vi "Update_DATA.vi"(8 "error in (no error)":errorcluster, 10 "Name":string, 11 "HIS in":refnum<class "HIS.lvclass">) -> (0 "error out":errorcluster, 3 "HIS out":refnum<class "HIS.lvclass">)   [LabVIEW 2015]
uses:
  HIS.lvclass
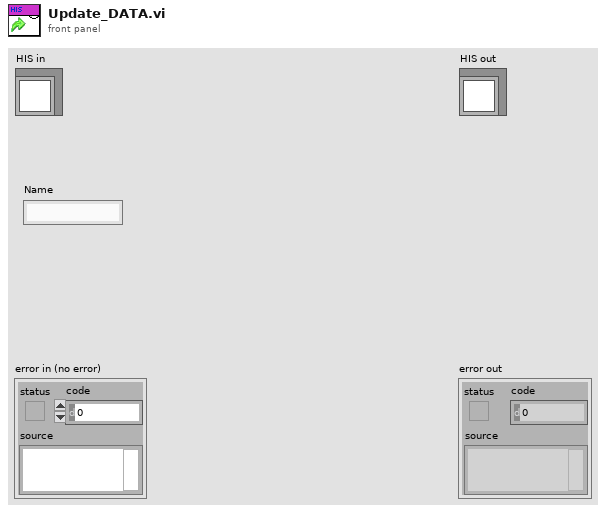
[diagram p1: front panel]
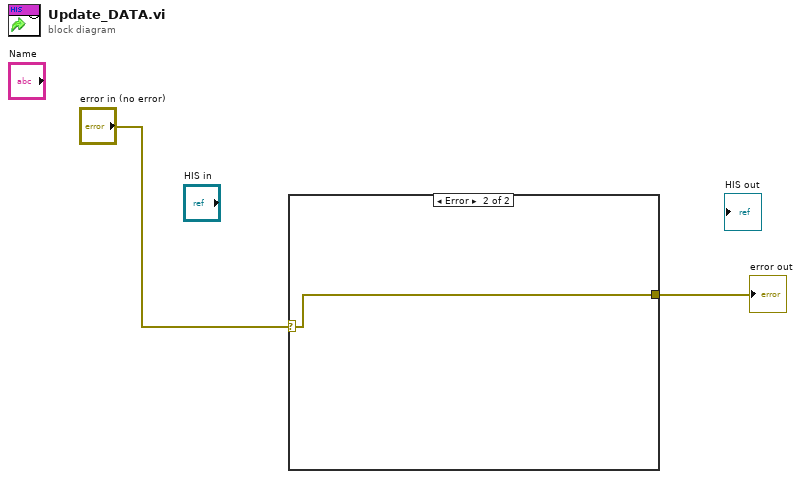
[diagram p0: block diagram]
diagram:
  n1 = case shown="Error" "error in (no error)" {
    selector: "error in (no error)" -> [_ w3]
    tunnel: [_ w3] -> w1
    frame No Error {
    }
    frame Error {
    }
  }
  "error out" <- w1
